vi "Extract Element.vi"(10 "index":i32, 11 "Priority Queue in":refnum<class "NI_Robotics_Priority Queue.lvclass">) -> (0 "node Ref":refnum<data-value>, 1 "g":dbl, 2 "f":dbl, 3 "Priority Queue out":refnum<class "NI_Robotics_Priority Queue.lvclass">)   [LabVIEW 2017, in "NI_Robotics_Priority Queue.lvclass"]
uses:
  <vilib>/robotics/Navigation/shared/Priority Queue/NI_Robotics_Priority Queue.lvclass
  <vilib>/robotics/Navigation/shared/MapNode/AbstractMapNode/NI_Robotics_AbstractMapNode.lvclass
  <vilib>/robotics/Navigation/shared/Priority Queue/NI_Robotics_Priority Queue.lvclass/NI_Robotics_Priority Queue.ctl
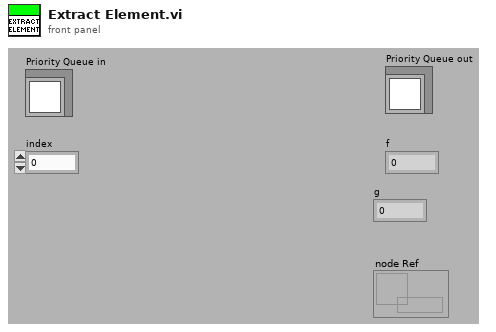
[diagram p1: front panel]
types:
  T1 = typedef "NI_Robotics_Priority Queue.lvclass/Open List Element.ctl" = cluster{"f":dbl, "g":dbl, "node Ref":refnum<data-value>}
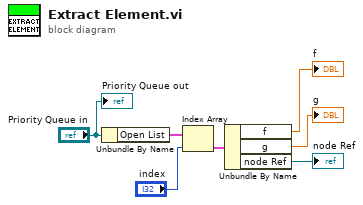
[diagram p0: block diagram]
diagram:
  n1 = Unbundle By Name("Priority Queue in") -> ("Open List"=w7:T1[])
  n2 = Index Array(array=w7, index="index") -> (element=w5:T1)
  n3 = Unbundle By Name(w5) -> ("f"=→"f":dbl, "g"=→"g":dbl, "node Ref"=→"node Ref":refnum<data-value>)
  "Priority Queue out" <- "Priority Queue in"
